vi "Get Autonomous Time Settings.vi"(11 "Autonomous Selectin":string="Robot Right Switch Left") -> (1 "Auto Time Calc Selected":T1(array[cluster]), 3 "Autonomous Data Selected":T2(array[cluster]))   [LabVIEW 2017]
uses:
  Framework/Robot Global Data.vi
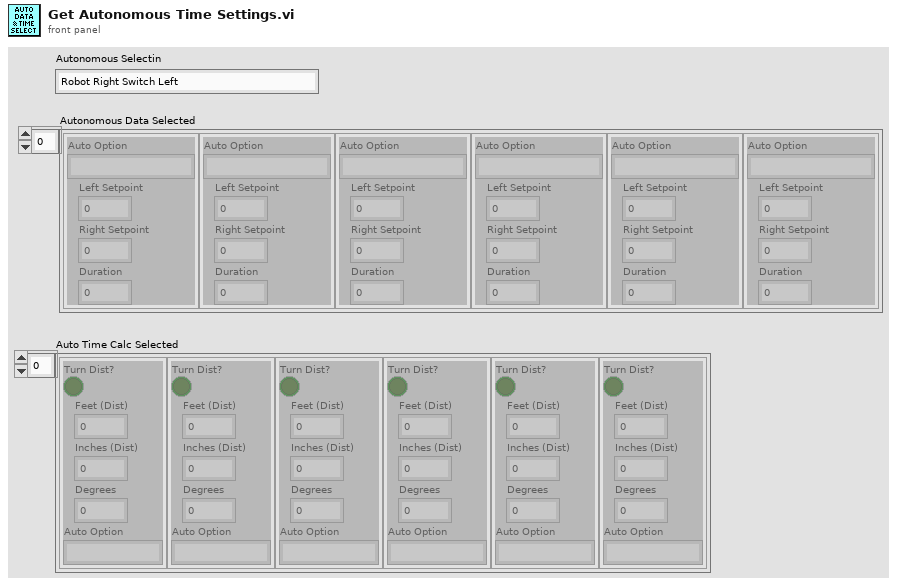
[diagram p1: front panel]
types:
  T1 = cluster{"Turn Dist?":bool, "Feet (Dist)":dbl, "Inches (Dist)":dbl, "Degrees":dbl, "Auto Option":string}[]
  T2 = cluster{"Auto Option":string, "Left Setpoint":dbl, "Right Setpoint":dbl, "Duration":dbl}[]
  T3 = cluster{"Auto Option":string, "Left Setpoint":dbl, "Right Setpoint":dbl, "Duration":dbl}[][]
  T4 = cluster{"Turn Dist?":bool, "Feet (Dist)":dbl, "Inches (Dist)":dbl, "Degrees":dbl, "Auto Option":string}[][]
  T5 = cluster{"Auto Option":string, "Left Setpoint":dbl, "Right Setpoint":dbl, "Duration":dbl}
  T6 = cluster{"Turn Dist?":bool, "Feet (Dist)":dbl, "Inches (Dist)":dbl, "Degrees":dbl, "Auto Option":string}
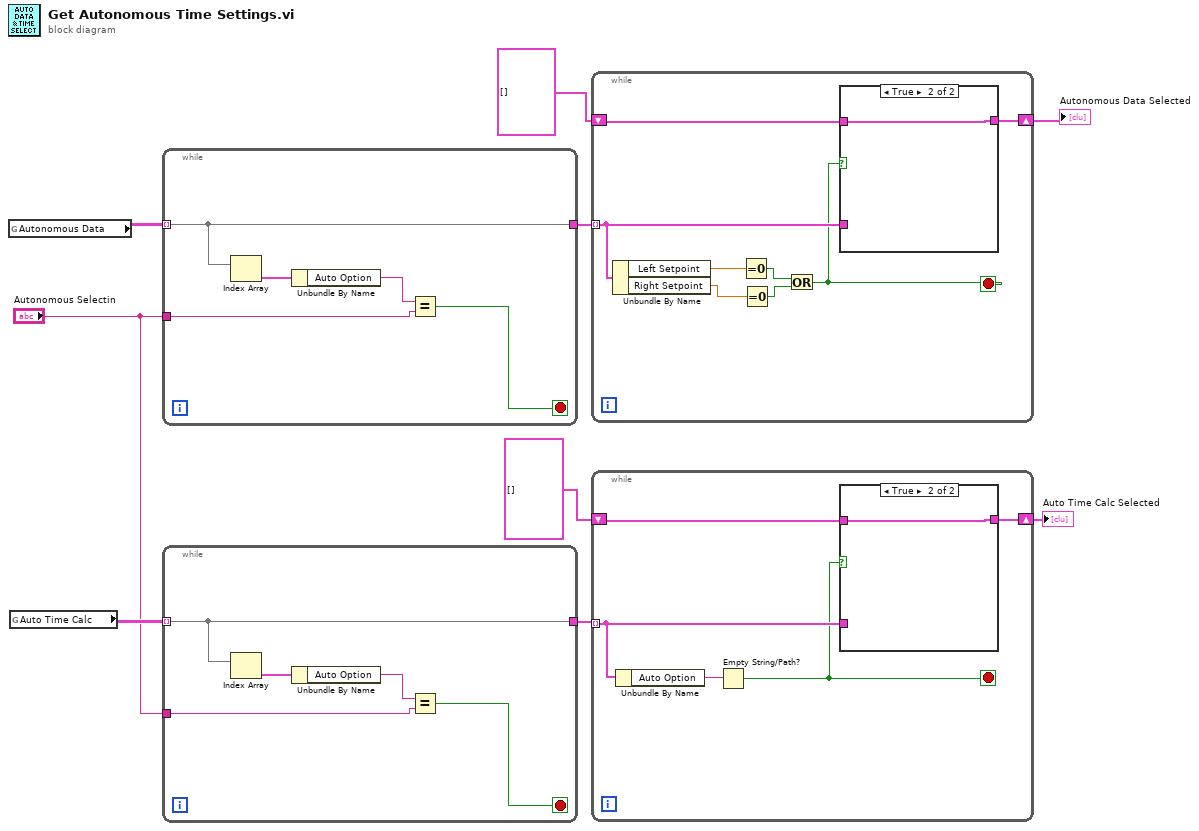
[diagram p0: block diagram]
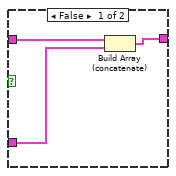
[diagram p2: hidden frame]
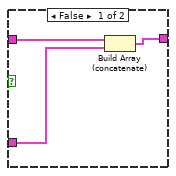
[diagram p3: hidden frame]
diagram:
  n1 = global read "Robot Global Data.vi" "Autonomous Data"() -> (w9:T3)
  n2 = global read "Robot Global Data.vi" "Auto Time Calc"() -> (w5:T4)
  n3 = while {
    tunnel: w9 -> [w10] mode=indexing
    tunnel: "Autonomous Selectin" -> [w12]
    tunnel: [w10] -> w8
    stop <- w11 stop-if-true
    n4 = Index Array(array=w10) -> (element=w14:T5)  [unwired: 1 in]
    n5 = Unbundle By Name(w14) -> ("Auto Option"=w13:string)
    n6 = Equal?(x=w13, y=w12) -> (x = y?=w11:bool)
  }
  n7 = while {
    tunnel: w5 -> [w15] mode=indexing
    tunnel: "Autonomous Selectin" -> [w17]
    tunnel: [w15] -> w3
    stop <- w16 stop-if-true
    n8 = Index Array(array=w15) -> (element=w19:T6)  [unwired: 1 in]
    n9 = Unbundle By Name(w19) -> ("Auto Option"=w18:string)
    n10 = Equal?(x=w18, y=w17) -> (x = y?=w16:bool)
  }
  n11 = while {
    tunnel: w8 -> [w22] mode=indexing
    shift-right: [w21] -> w6
    shift-left: T2 [] -> [w23]
    stop <- w20 stop-if-true
    n12 = Unbundle By Name(w22) -> ("Left Setpoint"=w27:dbl, "Right Setpoint"=w24:dbl)
    n13 = Equal To 0?(x=w27) -> (x = 0?=w25:bool)
    n14 = Equal To 0?(x=w24) -> (x = 0?=w26:bool)
    n15 = Or(x=w25, y=w26) -> (x .or. y?=w20:bool)
    n16 = case shown="True" w20 {
      tunnel: w23 -> [w30 w31]
      tunnel: w22 -> [w29 _]
      tunnel: [w28 w31] -> w21
      frame False {
        n17 = Build Array (concatenate)(w30, w29) -> (w28:T2)
      }
      frame True {
      }
    }
  }
  "Autonomous Data Selected" <- w6
  n18 = while {
    tunnel: w3 -> [w34] mode=indexing
    shift-right: [w35] -> w1
    shift-left: T1 [] -> [w36]
    stop <- w32 stop-if-true
    n19 = Unbundle By Name(w34) -> ("Auto Option"=w33:string)
    n20 = Empty String/Path?(string/path=w33) -> (empty?=w32:bool)
    n21 = case shown="True" w32 {
      tunnel: w36 -> [w39 w40]
      tunnel: w34 -> [w38 _]
      tunnel: [w37 w40] -> w35
      frame False {
        n22 = Build Array (concatenate)(w39, w38) -> (w37:T1)
      }
      frame True {
      }
    }
  }
  "Auto Time Calc Selected" <- w1
